vi "PLQY calculation.Final.vi"() -> ()   [LabVIEW 2020]
uses:
  <vilib>/Utility/file.llb/Read Delimited Spreadsheet (DBL).vi
  <vilib>/gmath/NI_Gmath.lvlib
  <vilib>/Analysis/NI_AALPro.lvlib
panel:
  in  "README":string="1: select Device > 2: select method > 3: set profile range for laser and PL peaks > 4: set time in second > 5: choose data path if not yet saved as constant in block diagram > 6: have fun\nQEpro: min=360nm & max =1100nm"
  out "PLQY with reabsorption":dbl
  out "PLQY without reabsorption":dbl
  out "laser loop number":i32
  in  "laser range end":dbl
  in  "laser range start":dbl
  out "PL loop number":i32
  in  "PL range start":dbl
  in  "PL range end":dbl
  out "Lb":dbl
  out "Pb":dbl
  out "Lc":dbl
  out "Pc":dbl
  out "La":dbl
  in  "Time(s) for Laser profile":dbl=0.1
  in  "Time(s) for PL profile":dbl=0.1
  in  "stop":bool
  out "Laser signal":cluster{"all rows":dbl[], "all rows":dbl[]}(graph)
  out "PL signal":cluster{"all rows":dbl[], "all rows":dbl[]}(graph)
  in  "Method":u16(ring) items=["3 step", "5 step"]
  out "DATA condition":string="No sample"
  in  "Device":u16(ring) items=["QE pro", "USB2000", "USB2000B"]
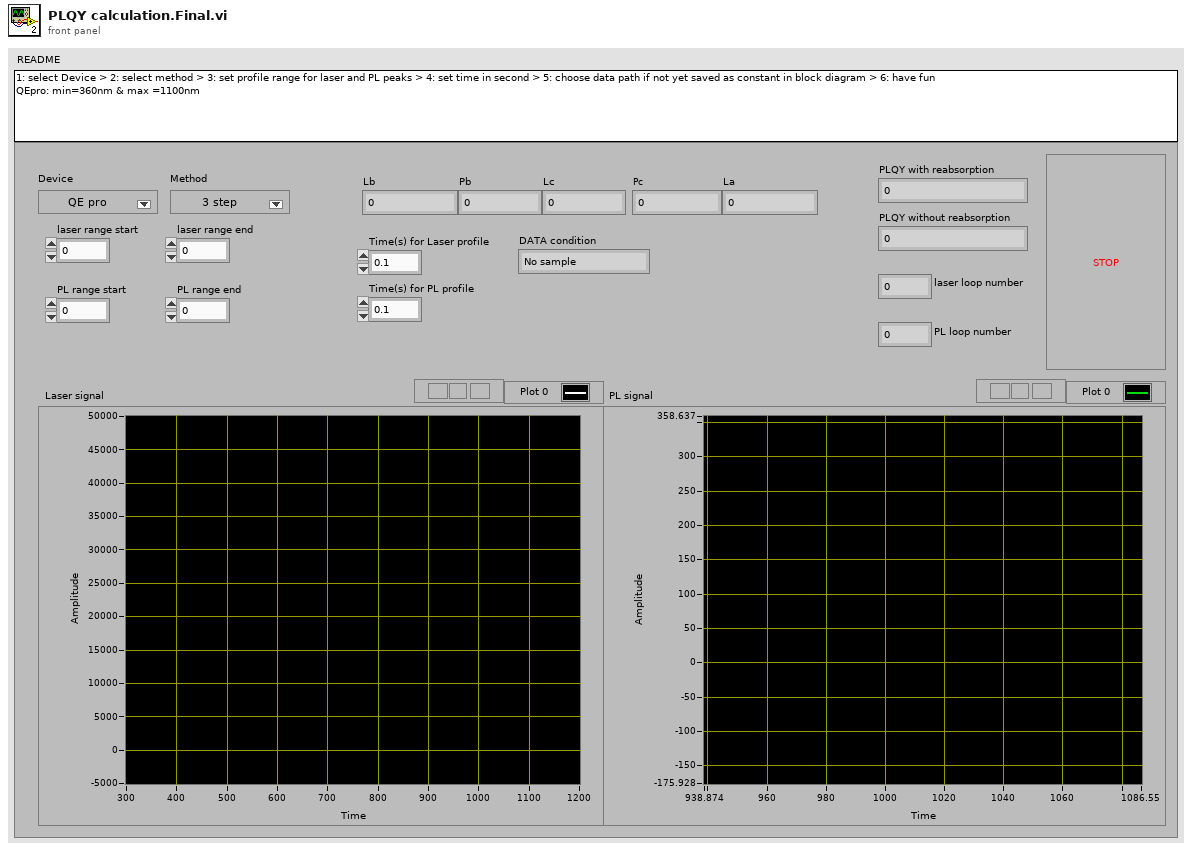
[diagram p1: front panel]
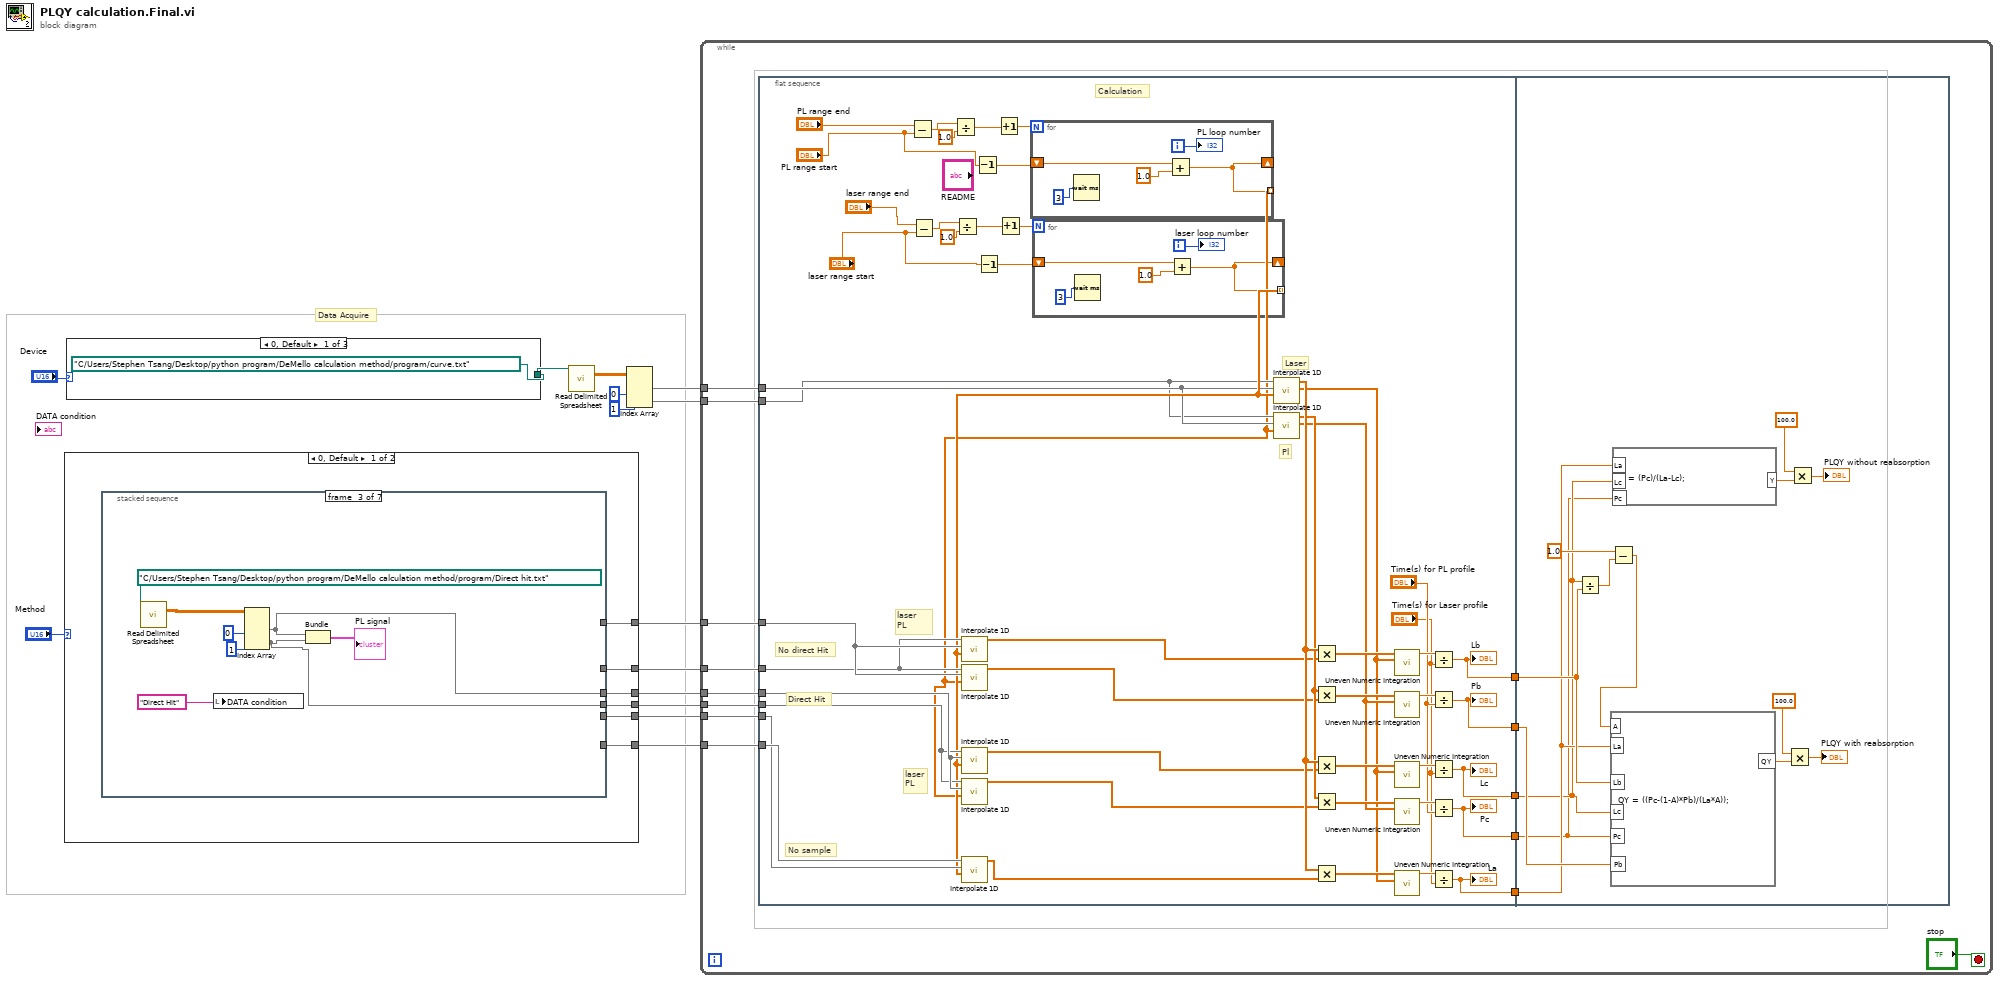
[diagram p0: block diagram]
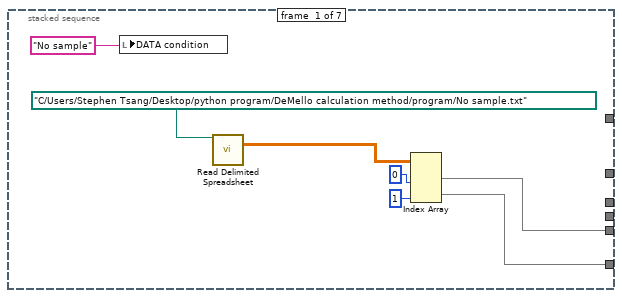
[diagram p2: hidden frame]
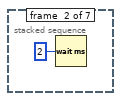
[diagram p3: hidden frame]
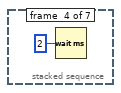
[diagram p4: hidden frame]
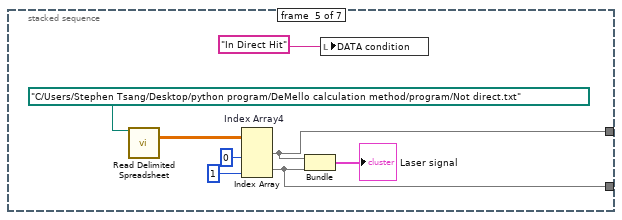
[diagram p5: hidden frame]
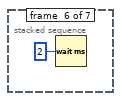
[diagram p6: hidden frame]
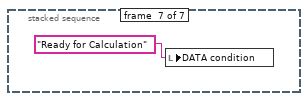
[diagram p7: hidden frame]
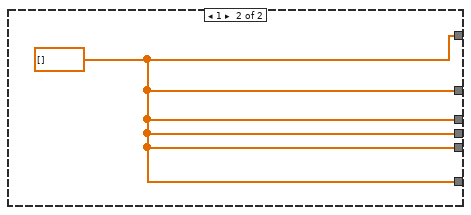
[diagram p8: hidden frame]
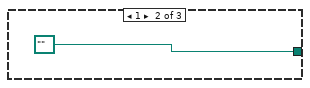
[diagram p9: hidden frame]
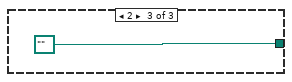
[diagram p10: hidden frame]
diagram:
  # "Data Acquire"
  n1 = case shown="0, Default" "Method" {
    tunnel: [w20 w48] -> w8
    tunnel: [w19 w48] -> w7
    tunnel: [w18 w48] -> w6
    tunnel: [w17 w48] -> w5
    tunnel: [w16 w48] -> w4
    tunnel: [w15 w48] -> w3
    frame 0, Default {
      n2 = stacked-sequence {
        tunnel: [w22 _ _ _ _ _ _] -> w20
        tunnel: [w21 _ _ _ _ _ _] -> w19
        tunnel: [_ _ w30 _ _ _ _] -> w18
        tunnel: [_ _ w29 _ _ _ _] -> w17
        tunnel: [_ _ _ _ w39 _ _] -> w16
        tunnel: [_ _ _ _ w38 _ _] -> w15
        frame #0 {
          n3 = local write "DATA condition"("No sample") -> ()
          n4 = call-poly <vilib>:"Read Delimited Spreadsheet.vi"("file path (dialog if empty)"=path "C:/Users/Stephen Tsang/Desktop/python program/DeMello calculation method/program/No sample.txt") -> ("all rows"=w25:dbl[][])  [unwired: 9 in, 5 out]
          n5 = Index Array "Index Array"(array=w25, index (col) #1=0 ("index"), index (col) #2=1 ("index (col)")) -> (element #1=w21:dbl[], element #2=w22:dbl[])  [unwired: 2 in]
        }
        frame #1 {
          n6 = Wait (ms)(milliseconds to wait=u32 2) -> ()  [unwired: 1 out]
        }
        frame #2 {
          n7 = call-poly <vilib>:"Read Delimited Spreadsheet.vi"("file path (dialog if empty)"=path "C:/Users/Stephen Tsang/Desktop/python program/DeMello calculation method/program/Direct hit.txt") -> ("all rows"=w34:dbl[][])  [unwired: 9 in, 5 out]
          n8 = local write "DATA condition"("Direct Hit") -> ()
          n9 = Index Array "Index Array"(array=w34, index (col) #1=0 ("index"), index (col) #2=1 ("index (col)")) -> (element #1=w30:dbl[], element #2=w29:dbl[])  [unwired: 2 in]
          n10 = Bundle("all rows"=w30, "all rows"=w29) -> (→"PL signal":cluster{"all rows":dbl[], "all rows":dbl[]})  [unwired: 1 in]
        }
        frame #3 {
          n11 = Wait (ms)(milliseconds to wait=u32 2) -> ()  [unwired: 1 out]
        }
        frame #4 {
          n12 = call-poly <vilib>:"Read Delimited Spreadsheet.vi"("file path (dialog if empty)"=path "C:/Users/Stephen Tsang/Desktop/python program/DeMello calculation method/program/Not direct.txt") -> ("all rows"=w43:dbl[][])  [unwired: 9 in, 5 out]
          n13 = Index Array "Index Array4"(array=w43, index (col) #1=0 ("index"), index (col) #2=1 ("index (col)")) -> (element #1=w39:dbl[], element #2=w38:dbl[])  [unwired: 2 in]
          n14 = Bundle("all rows"=w39, "all rows"=w38) -> (→"Laser signal":cluster{"all rows":dbl[], "all rows":dbl[]})  [unwired: 1 in]
          n15 = local write "DATA condition"("In Direct Hit") -> ()
        }
        frame #5 {
          n16 = Wait (ms)(milliseconds to wait=u32 2) -> ()  [unwired: 1 out]
        }
        frame #6 {
          n17 = local write "DATA condition"("Ready for Calculation" ("DATA inputing")) -> ()
        }
      }
    }
    frame 1 {
      w48 = dbl[] [] ("all rows")
    }
  }
  n18 = case shown="0, Default" "Device" {
    tunnel: [path "C:/Users/Stephen Tsang/Desktop/python program/DeMello calculation method/program/curve.txt" ("file path (dialog if empty)") path "" ("file path (dialog if empty)") path "" ("file path (dialog if empty)")] -> w12
    frame 0, Default {
    }
    frame 1 {
    }
    frame 2 {
    }
  }
  n19 = call-poly <vilib>:"Read Delimited Spreadsheet.vi"("file path (dialog if empty)"=w12) -> ("all rows"=w11:dbl[][])  [unwired: 9 in, 5 out]
  n20 = Index Array "Index Array"(array=w11, index (col) #1=0 ("disabled index (col)"), index (col) #2=1 ("index (col)")) -> (element #1=w2:dbl[], element #2=w1:dbl[])  [unwired: 2 in]
  n21 = while {
    tunnel: w8 -> [w60]
    tunnel: w7 -> [w59]
    tunnel: w6 -> [w58]
    tunnel: w5 -> [w57]
    tunnel: w4 -> [w56]
    tunnel: w3 -> [w55]
    tunnel: w2 -> [w54]
    tunnel: w1 -> [w53]
    stop <- "stop" stop-if-true
    n22 = flat-sequence {
      tunnel: w60 -> [w110]
      tunnel: w59 -> [w100]
      tunnel: w58 -> [w99]
      tunnel: w57 -> [w98]
      tunnel: w56 -> [w97]
      tunnel: w55 -> [w96]
      tunnel: w54 -> [w94]
      tunnel: w53 -> [w93]
      tunnel: [w70] -> w65
      tunnel: [w69] -> w64
      tunnel: [w68] -> w63
      tunnel: [w67] -> w62
      tunnel: [w66] -> w61
      tunnel: w65 -> [w131]
      tunnel: w64 -> [w129]
      tunnel: w63 -> [w130]
      tunnel: w62 -> [w139]
      tunnel: w61 -> [w137]
      frame #0 {
        # "Calculation"
        # "Pl"
        # "Laser"
        # "laser\nPL"
        # "laser\nPL"
        # "No direct Hit"
        # "Direct Hit"
        # "No sample"
        n23 = Subtract(x="PL range end", y="PL range start") -> (x-y=w107:dbl)
        n24 = Subtract(x="laser range end", y="laser range start") -> (x-y=w115:dbl)
        n25 = Divide(x=w107, y=1.0) -> (x/y=w105:dbl)
        n26 = Divide(x=w115, y=1.0) -> (x/y=w113:dbl)
        n27 = Decrement(x="PL range start") -> (x-1=w103:dbl)
        n28 = Decrement(x="laser range start") -> (x-1=w111:dbl)
        n29 = Increment(x=w105) -> (x+1=w104:dbl)
        n30 = Increment(x=w113) -> (x+1=w112:dbl)
        n31 = for {
          N: w104 -> [_]
          shift-right: [w116] -> _
          shift-left: w103 -> [w117]
          tunnel: [w116] -> w85 mode=indexing
          i -> [w119]
          n32 = Wait (ms)(milliseconds to wait=u32 3) -> ()  [unwired: 1 out]
          n33 = Add(x=w117, y=1.0) -> (x+y=w116:dbl)
          "PL loop number" <- w119
        }
        n34 = call <vilib>:"Interpolate 1D.vi"("xi"=w85, "X"=w97, "Y"=w96) -> ("yi"=w86:dbl[])  [unwired: 6 in, 2 out]
        n35 = call <vilib>:"Interpolate 1D.vi"("xi"=w85, "X"=w99, "Y"=w98) -> ("yi"=w88:dbl[])  [unwired: 6 in, 2 out]
        n36 = for {
          N: w112 -> [_]
          shift-right: [w121] -> _
          shift-left: w111 -> [w122]
          tunnel: [w121] -> w95 mode=indexing
          i -> [w124]
          n37 = Wait (ms)(milliseconds to wait=u32 3) -> ()  [unwired: 1 out]
          n38 = Add(x=w122, y=1.0) -> (x+y=w121:dbl)
          "laser loop number" <- w124
        }
        n39 = call <vilib>:"Interpolate 1D.vi"("xi"=w95, "X"=w97, "Y"=w96) -> ("yi"=w87:dbl[])  [unwired: 6 in, 2 out]
        n40 = call <vilib>:"Interpolate 1D.vi"("xi"=w95, "X"=w99, "Y"=w98) -> ("yi"=w89:dbl[])  [unwired: 6 in, 2 out]
        n41 = call <vilib>:"Interpolate 1D.vi"("xi"=w95, "X"=w100, "Y"=w110) -> ("yi"=w92:dbl[])  [unwired: 6 in, 2 out]
        n42 = call <vilib>:"Interpolate 1D.vi"("xi"=w95, "X"=w94, "Y"=w93) -> ("xi used"=w78:dbl[], "yi"=w91:dbl[])  [unwired: 6 in, 1 out]
        n43 = call <vilib>:"Interpolate 1D.vi"("xi"=w85, "X"=w94, "Y"=w93) -> ("xi used"=w79:dbl[], "yi"=w90:dbl[])  [unwired: 6 in, 1 out]
        n44 = Multiply(x=w91, y=w87) -> (x*y=w80:dbl[])
        n45 = Multiply(x=w90, y=w86) -> (x*y=w81:dbl[])
        n46 = Multiply(x=w91, y=w89) -> (x*y=w82:dbl[])
        n47 = Multiply(x=w90, y=w88) -> (x*y=w83:dbl[])
        n48 = Multiply(x=w91, y=w92) -> (x*y=w84:dbl[])
        n49 = call <vilib>:"Uneven Numeric Integration.vi"("T"=w78, "X"=w80) -> ("result"=w73:dbl)  [unwired: 8 in, 1 out]
        n50 = call <vilib>:"Uneven Numeric Integration.vi"("T"=w79, "X"=w81) -> ("result"=w74:dbl)  [unwired: 8 in, 1 out]
        n51 = call <vilib>:"Uneven Numeric Integration.vi"("T"=w78, "X"=w82) -> ("result"=w75:dbl)  [unwired: 8 in, 1 out]
        n52 = call <vilib>:"Uneven Numeric Integration.vi"("T"=w79, "X"=w83) -> ("result"=w76:dbl)  [unwired: 8 in, 1 out]
        n53 = call <vilib>:"Uneven Numeric Integration.vi"("T"=w78, "X"=w84) -> ("result"=w77:dbl)  [unwired: 8 in, 1 out]
        n54 = Divide(x=w73, y="Time(s) for Laser profile") -> (x/y=w66:dbl)
        "Lb" <- w66
        n55 = Divide(x=w74, y="Time(s) for PL profile") -> (x/y=w67:dbl)
        "Pb" <- w67
        n56 = Divide(x=w75, y="Time(s) for Laser profile") -> (x/y=w68:dbl)
        "Lc" <- w68
        n57 = Divide(x=w76, y="Time(s) for PL profile") -> (x/y=w69:dbl)
        "Pc" <- w69
        n58 = Divide(x=w77, y="Time(s) for Laser profile") -> (x/y=w70:dbl)
        "La" <- w70
      }
      frame #1 {
        n59 = Divide(x=w130, y=w137) -> (x/y=w136:dbl)
        n60 = Subtract(x=1.0, y=w136) -> (x-y=w135:dbl)
        n61 = formula code="QY = ((Pc-(1-A)*Pb)/(La*A));"("La"=w131, "Lb"=w137, "Lc"=w130, "Pc"=w129, "Pb"=w139, "A"=w135) -> ("QY"=w133:dbl)
        n62 = formula code="Y = (Pc)/(La-Lc);"("La"=w131, "Lc"=w130, "Pc"=w129) -> ("Y"=w126:dbl)
        n63 = Multiply(x=100.0, y=w133) -> (x*y=→"PLQY with reabsorption":dbl)
        n64 = Multiply(x=100.0, y=w126) -> (x*y=→"PLQY without reabsorption":dbl)
      }
    }
  }
